vi "AT Register Feature Callback A.vi"(8 "error in (no error)":errorcluster, 10 "Feature":string, 11 "Handle":i32) -> (0 "error out":errorcluster, 1 "Event":refnum<user-event>, 2 "Event Registration Refnum":refnum<event-registration>, 3 "Status":i32)   [LabVIEW 2009]
doc: "Register Feature Callback\n\nOutput:\n I32 Status\n EventRegistrationRefnum Event Registration Refnum\n Event Event\n\nParameters:\n I32 Handle\n String Feature\n\nDescription\nTo retrieve a notification each time the value or other properties of a feature changes you can use this function to register a callback event. The Feature that you wish to receive notifications for is passed into the function. The context parameter is the same as that used when registering the callback and is sent unmodified. \nAs soon as this callback is registered a single callback will be made immediately to allow the callback handling code to perform any Initialisation code to set up monitoring of the feature."
uses:
  atlvcallbacks.dll
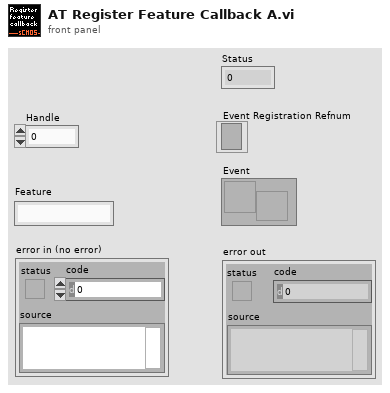
[diagram p1: front panel]
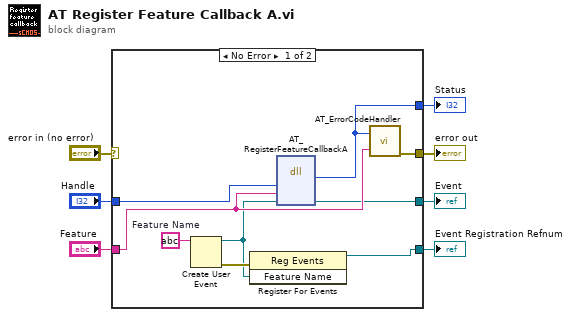
[diagram p0: block diagram]
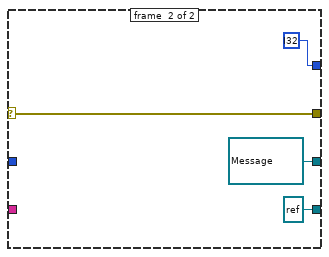
[diagram p2: hidden frame]
diagram:
  n1 = case shown="No Error" "error in (no error)" {
    selector: "error in (no error)" -> [_ w20]
    tunnel: "Feature" -> [w14 _]
    tunnel: "Handle" -> [w16 _]
    tunnel: [w15 i32 ? ("Status")] -> w4
    tunnel: [w13 w20] -> w3
    tunnel: [w9 refnum<event-registration> ? ("Event Registration Refnum")] -> w1
    tunnel: [w8 refnum<user-event> ? ("Event")] -> w2
    frame #0 {
      w12 = string ?  # Feature Name
      n2 = Create User Event(user event datatype=w12) -> (user event=w10:refnum<user-event>, error out=w11:errorcluster)  [unwired: 1 in]
      n3 = register-events(error in=w11, w10) -> (reference out=w9:refnum<event-registration>)  [unwired: 1 in, 1 out]
      n4 = dll-call lib="atlvcallbacks.dll" fn="AT_RegisterFeatureCallbackA"("Handle"=w16, "Feature"=w14, "Event"=w10) -> ("Status"=w15:i32, "Event"=w8:refnum<user-event>)  [unwired: 5 in, 2 out]
      n5 = call "AT_ErrorCodeHandler.vi"("Error"=w15, "Feature Name"=w14) -> ("error out"=w13:errorcluster)  [unwired: 5 in]
    }
    frame #1 {
    }
  }
  "error out" <- w3
  "Status" <- w4
  "Event" <- w2
  "Event Registration Refnum" <- w1
